vi "T Vector Predictive Filter.vi"(6 "threshold":dbl=0.0625 format="%#_13g", 9 "Tag ID":i32, 10 "t Translation Vector":dbl[](array[numeric]) format="%#.6f") -> (2 "t Translation Vector Prodictive filtered":dbl[](array[numeric]))   [LabVIEW 2025]
panel:
  out "Predictive Filtered Data":dbl[][](array[numeric])
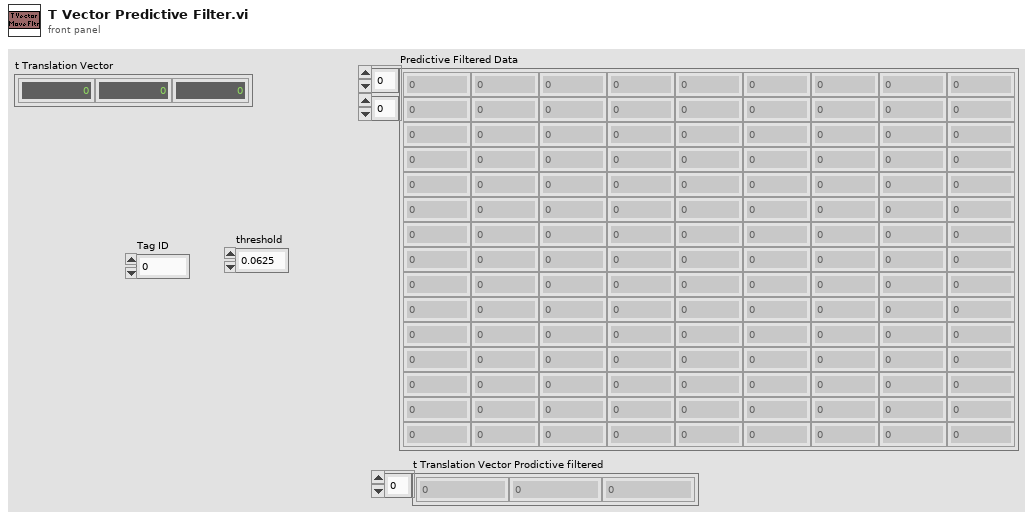
[diagram p1: front panel]
types:
  T1 = cluster{"Previous Position ":dbl[][], "Filter Factor a":dbl[], "Velocity Previous":dbl[][], "Filter Factor ß":dbl[]}
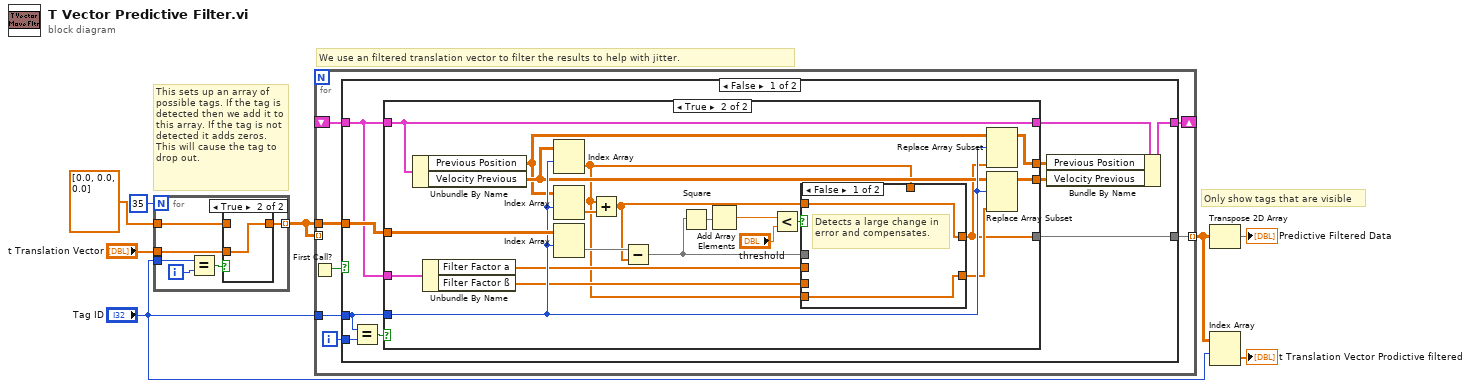
[diagram p0: block diagram]
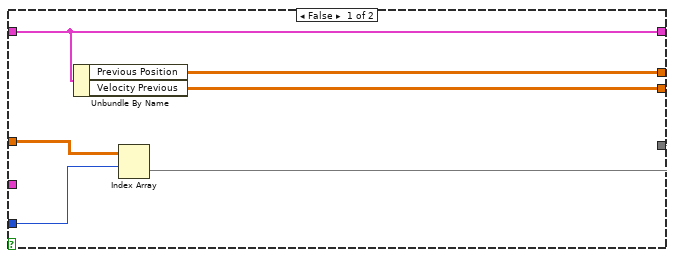
[diagram p2: hidden frame]
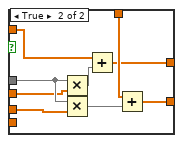
[diagram p3: hidden frame]
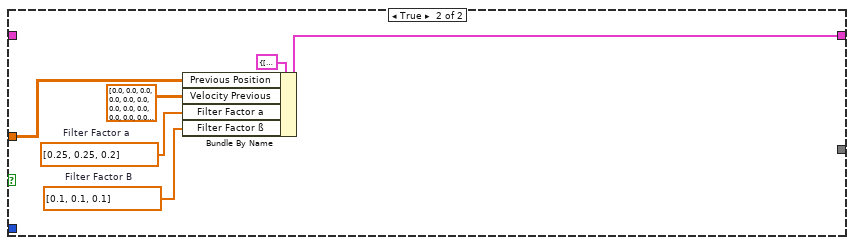
[diagram p4: hidden frame]
diagram:
  # "Only show tags that are visible"
  # "We use an filtered translation vector to filter the results to help with jitter."
  # "This sets up an array of possible tags. If the tag is detected then we add it to this array. If the tag is not detected it adds zeros. This will cause the tag to drop out."
  n1 = for {
    N: 35 -> [_]
    tunnel: dbl[] [0.0, 0.0, 0.0] ("f") -> [w14]
    tunnel: "t Translation Vector" -> [w9]
    tunnel: [w13] -> w5 mode=indexing
    tunnel: "Tag ID" -> [w11]
    i -> [w12]
    n2 = Equal?(x=w11, y=w12) -> (x = y?=w10:bool)
    n3 = case shown="True" w10 {
      tunnel: w9 -> [_ w16]
      tunnel: [w15 w16] -> w13
      tunnel: w14 -> [w15 _]
      frame False {
      }
      frame True {
      }
    }
  }
  n4 = for {
    shift-right: [w23] -> _
    shift-left: _ -> [w21]
    tunnel: [w20] -> w2 mode=indexing
    tunnel: w5 -> [w22]
    tunnel: "Tag ID" -> [w18]
    tunnel: w5 -> [_] mode=indexing
    i -> [w19]
    n5 = First Call?() -> (First Call?: T/F=w17:bool)
    n6 = case shown="False" w17 {
      tunnel: [w33 w76] -> w23
      tunnel: w22 -> [w32 w74]
      tunnel: w21 -> [w31 _]
      tunnel: [w30 _] -> w20
      tunnel: w19 -> [w25 _]
      tunnel: w18 -> [w24 _]
      frame False {
        n7 = Equal?(x=w24, y=w25) -> (x = y?=w27:bool)
        n8 = case shown="True" w27 {
          tunnel: w32 -> [w39 w59]
          tunnel: w31 -> [_ w60]
          tunnel: [w37 w51] -> w30
          tunnel: w24 -> [w38 w55]
          tunnel: w31 -> [w36 w58]
          tunnel: [w36 w58] -> w29
          tunnel: [w34 w57] -> w28
          tunnel: [w35 w56] -> w26
          frame False {
            n9 = Unbundle By Name(w36) -> ("Previous Position"=w35:dbl[][], "Velocity Previous"=w34:dbl[][])
            n10 = Index Array(array=w39, index (row)=w38) -> (element=w37:dbl[])  [unwired: 1 in]
          }
          frame True {
            n11 = Unbundle By Name(w58) -> ("Previous Position"=w47:dbl[][], "Velocity Previous"=w54:dbl[][])
            n12 = Unbundle By Name(w60) -> ("Filter Factor a"=w50:dbl[], "Filter Factor ß"=w49:dbl[])
            n13 = Index Array(array=w54, index (row)=w55) -> (element=w41:dbl[])  [unwired: 1 in]
            n14 = Index Array(array=w47, index (row)=w55) -> (element=w44:dbl[])  [unwired: 1 in]
            n15 = Index Array(array=w59, index (row)=w55) -> (element=w53:dbl[])  [unwired: 1 in]
            n16 = Add(x=w41, y=w44) -> (x+y=w48:dbl[])
            n17 = Subtract(x=w53, y=w48) -> (x-y=w46:dbl[])
            n18 = Square(x=w46) -> (x^2=w45:dbl[])
            n19 = Add Array Elements(numeric array=w45) -> (sum=w40:dbl)
            n20 = Less?(x=w40, y="threshold") -> (x < y?=w42:bool)
            n21 = case shown="False" w42 {
              tunnel: w41 -> [_ w71]
              tunnel: w46 -> [_ w70]
              tunnel: [w62 w68] -> w52
              tunnel: [w61 w67] -> w51
              tunnel: w50 -> [_ w66]
              tunnel: w49 -> [_ w65]
              tunnel: w48 -> [w61 w64]
              tunnel: w41 -> [w62 _]
              frame False {
                # "Detects a large change in error and compensates."
              }
              frame True {
                n22 = Multiply(x=w70, y=w66) -> (x*y=w63:dbl[])
                n23 = Multiply(x=w70, y=w65) -> (x*y=w69:dbl[])
                n24 = Add(x=w64, y=w63) -> (x+y=w67:dbl[])
                n25 = Add(x=w71, y=w69) -> (x+y=w68:dbl[])
              }
            }
            n26 = Replace Array Subset(array=w47, new element=w51, index (row)=w55) -> (w56:dbl[][])  [unwired: 1 in]
            n27 = Replace Array Subset(array=w54, new element=w52, index (row)=w55) -> (w57:dbl[][])  [unwired: 1 in]
          }
        }
        n28 = Bundle By Name(cluster=w29, "Previous Position"=w26, "Velocity Previous"=w28) -> (w33:T1)
      }
      frame True {
        w72 = dbl[] [0.1, 0.1, 0.1]  # Filter Factor B
        w73 = dbl[] [0.25, 0.25, 0.2]  # Filter Factor a
        n29 = Bundle By Name(cluster=T1 {"Previous Position "=[], "Filter Factor a"=[0.25, 0.25, 0.2], "Velocity Previous"=[], "Filter Factor ß"=[0.1, 0.1, 0.1]}, "Previous Position"=w74, "Velocity Previous"=dbl[][] [[0.0, 0.0, 0.0, 0.0], [0.0, 0.0, 0.0, 0.0], [0.0, 0.0, 0.0, 0.0], [0.0, 0.0, 0.0, 0.0], [0.0, 0.0, 0.0, 0.0], [0.0, 0.0, 0.0, 0.0], [0.0, 0.0, 0.0, 0.0], [0.0, 0.0, 0.0, 0.0], [0.0, 0.0, 0.0, 0.0], [0.0, 0.0, 0.0, 0.0], [0.0, 0.0, 0.0, 0.0], [0.0, 0.0, 0.0, 0.0], [0.0, 0.0, 0.0, 0.0], [0.0, 0.0, 0.0, 0.0], [0.0, 0.0, 0.0, 0.0], [0.0, 0.0, 0.0, 0.0], [0.0, 0.0, 0.0, 0.0], [0.0, 0.0, 0.0, 0.0], [0.0, 0.0, 0.0, 0.0], [0.0, 0.0, 0.0, 0.0], [0.0, 0.0, 0.0, 0.0], [0.0, 0.0, 0.0, 0.0], [0.0, 0.0, 0.0, 0.0], [0.0, 0.0, 0.0, 0.0], [0.0, 0.0, 0.0, 0.0], [0.0, 0.0, 0.0, 0.0], [0.0, 0.0, 0.0, 0.0], [0.0, 0.0, 0.0, 0.0], [0.0, 0.0, 0.0, 0.0], [0.0, 0.0, 0.0, 0.0], [0.0, 0.0, 0.0, 0.0], [0.0, 0.0, 0.0, 0.0], [0.0, 0.0, 0.0, 0.0], [0.0, 0.0, 0.0, 0.0], [0.0, 0.0, 0.0, 0.0], [0.0, 0.0, 0.0, 0.0]], "Filter Factor a"=w73, "Filter Factor ß"=w72) -> (w76:T1)
      }
    }
  }
  n30 = Transpose 2D Array(2D array=w2) -> (transposed array=→"Predictive Filtered Data":dbl[][])
  n31 = Index Array(array=w2, index (row)="Tag ID") -> (element=→"t Translation Vector Prodictive filtered":dbl[])  [unwired: 1 in]
